vi "Check for new data.vi"(0 "New Value FIFO":refnum<k33>, 1 "Interpolate Info In":T2 {"Interpolate Options"."method" items=["nearest", "linear", "spline", "cubic Hermite", "Lagrange"]}, 5 "Command FIFO":refnum<k33>, 7 "Load New Data?":dbl, 11 "error in (no error)":errorcluster) -> (3 "Interpolate Info Out":T2 {"Interpolate Options"."method" items=["nearest", "linear", "spline", "cubic Hermite", "Lagrange"]}, 6 "New Data Ready?":bool, 15 "error out":errorcluster)   [LabVIEW 2011, in "Interpolate 1D Array Custom Device.lvlib"]
doc: "Checks the 'New Data' Channel, and launches the sequence for the spreadsheet to be re-read by the asynchronous VI and bring back the new values."
uses:
  Interpolate 1D Array Custom Device.lvlib
  Interpolate Options.ctl
  <vilib>/ptbypt/NI_PtbyPt.lvlib
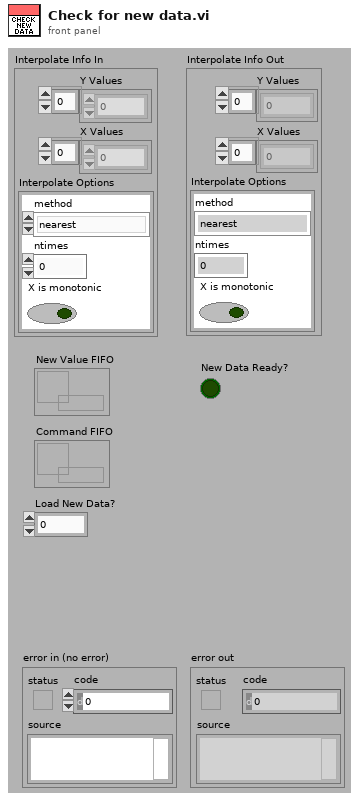
[diagram p1: front panel]
types:
  T1 = typedef "Interpolate 1D Array Custom Device.lvlib/Interpolate Options.ctl" = cluster{"method":i32, "ntimes":i32, "X is monotonic":bool}
  T2 = cluster{"Y Values":dbl[], "X Values":dbl[], "Interpolate Options":T1}
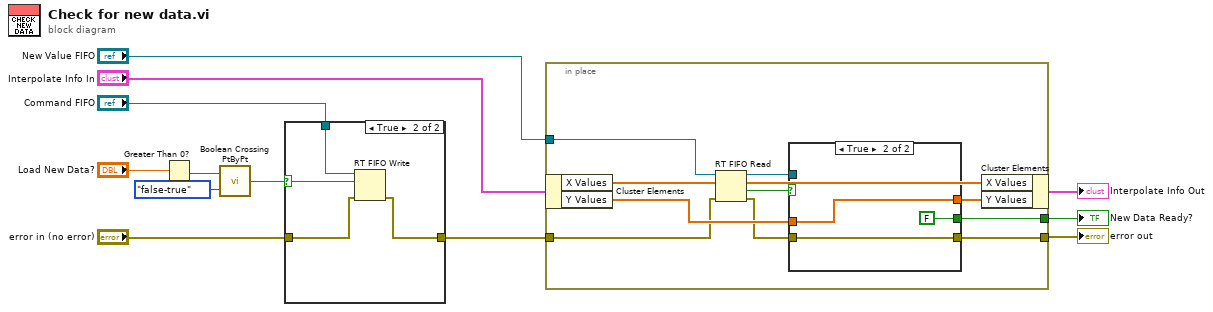
[diagram p0: block diagram]
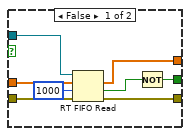
[diagram p2: hidden frame]
diagram:
  n1 = Greater Than 0?(x="Load New Data?") -> (x > 0?=w2:bool)
  n2 = call <vilib>:"Boolean Crossing PtByPt.vi"("direction"=enum16{"either", "false-true", "true-false"}."false-true", "input"=w2) -> ("crossing"=w1:bool)  [unwired: 1 in]
  n3 = case shown="True" w1 {
    selector: w1 -> [_ w16]
    tunnel: "Command FIFO" -> [_ w17]
    tunnel: "error in (no error)" -> [w13 w15]
    tunnel: [w13 w14] -> w7
    frame False {
    }
    frame True {
      n4 = RT FIFO Write(0:w17, 1:w16, 3:w15) -> (11:w14:errorcluster)  [unwired: 2 in, 3 out]
    }
  }
  n5 = in-place {
    in-place-border: "New Value FIFO" -> [w28]
    in-place-border: [w21] -> w6
    in-place-border: w7 -> [w20]
    in-place-border: [w18] -> w4
    n6 = in-place-cluster #1("Interpolate Info In") -> ("X Values"=w27:dbl[], "Y Values"=w24:dbl[])
    n7 = RT FIFO Read(0:w28, 1:w27, 3:w20) -> (8:w25:refnum<k33>, 9:w26:dbl[], 10:w19:bool, 11:w22:errorcluster)  [unwired: 1 in, 1 out]
    n8 = case shown="True" w19 {
      tunnel: w25 -> [w36 _]
      tunnel: w24 -> [w35 w39]
      tunnel: [w34 w39] -> w23
      tunnel: w22 -> [w33 w38]
      tunnel: [w32 w38] -> w21
      tunnel: [w30 FALSE] -> w18
      frame False {
        n9 = RT FIFO Read(0:w36, 1:w35, 2:1000 ("timeout in ms (0)"), 3:w33) -> (9:w34:dbl[], 10:w29:bool, 11:w32:errorcluster)  [unwired: 2 out]
        n10 = Not(x=w29) -> (.not. x?=w30:bool)
      }
      frame True {
      }
    }
    n11 = in-place-cluster #1("X Values"=w26, "Y Values"=w23) -> (→"Interpolate Info Out":T2)
  }
  "error out" <- w6
  "New Data Ready?" <- w4
